vi "_Save_data.vi"(0 "vihlp Path":path, 7 "Info extracted from old HTML":T1={"_vi_name_"="", "_vi_description_text_"="", "_vi_controls_and_indicators_descriptions_"="", "_name_of_owning_library_"="", "_owning_library_html_"="", "_Packages_"="Base Package", "_Platforms_"="Windows", "_details_text_"="Put details here", "_example_screenshot_"="", "_example_vi_"="", "_path_to_example_file_"=path "", "IsDetailsON?"=FALSE, "IsOwningLibraryON?"=FALSE, "IsExamplesON?"=FALSE, "IsTableON?"=FALSE, "IsScrollableON?"=FALSE, "IsDetailedHelpLinkON?"=FALSE, "Table Objects array"=[], "Table Descriptions array"=[], "Table Links array"=[], "Start path location"=enum."VI folder"}, 11 "error in":errorcluster) -> (15 "error out":errorcluster)   [LabVIEW 2012]
uses:
  _Controls and TypeDefs/InfoFromOldHTML_cluster.ctl
  _Controls and TypeDefs/StartPathLocation_enum.ctl
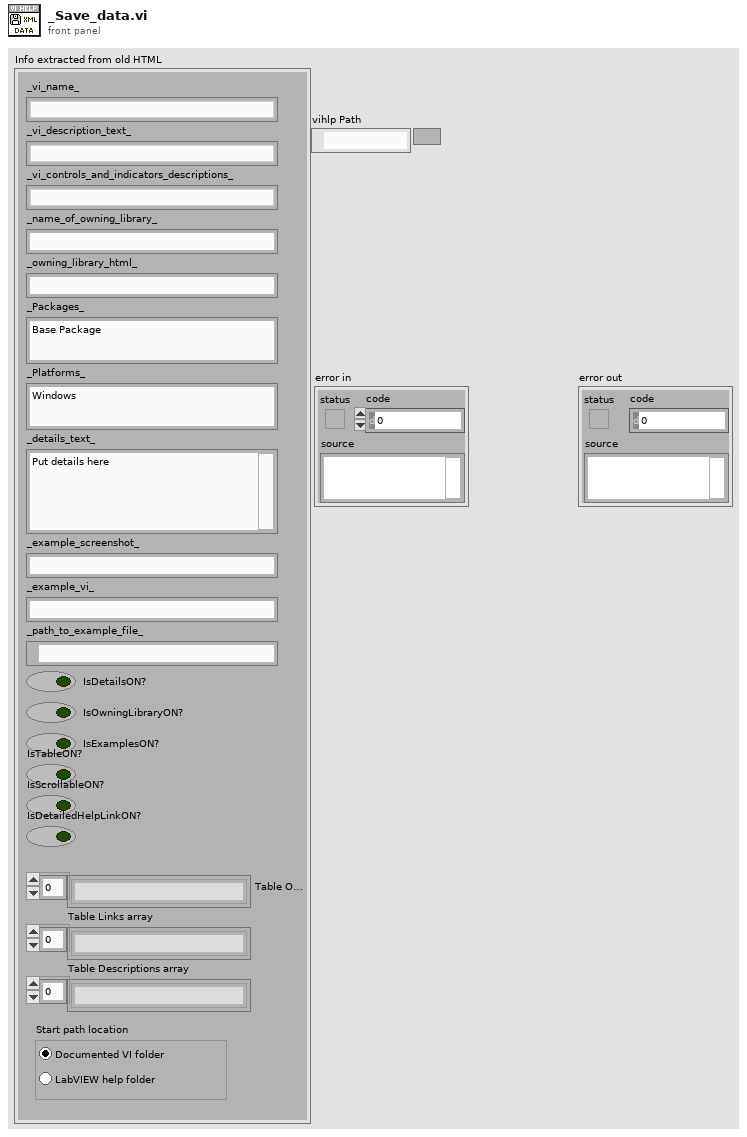
[diagram p1: front panel]
types:
  T1 = typedef "InfoFromOldHTML_cluster.ctl" = cluster{"_vi_name_":string, "_vi_description_text_":string, "_vi_controls_and_indicators_descriptions_":string, "_name_of_owning_library_":string, "_owning_library_html_":string, "_Packages_":string, "_Platforms_":string, "_details_text_":string, "_example_screenshot_":string, "_example_vi_":string, "_path_to_example_file_":path, "IsDetailsON?":bool, "IsOwningLibraryON?":bool, "IsExamplesON?":bool, "IsTableON?":bool, "IsScrollableON?":bool, "IsDetailedHelpLinkON?":bool, "Table Objects array":string[], "Table Descriptions array":string[], "Table Links array":string[], "Start path location":T2}
  T2 = typedef "StartPathLocation_enum.ctl" = enum32{"VI folder", "Help folder"}
  T3 = enum16{"open", "replace", "create", "open or create", "replace or create", "replace or create with confirmation"}
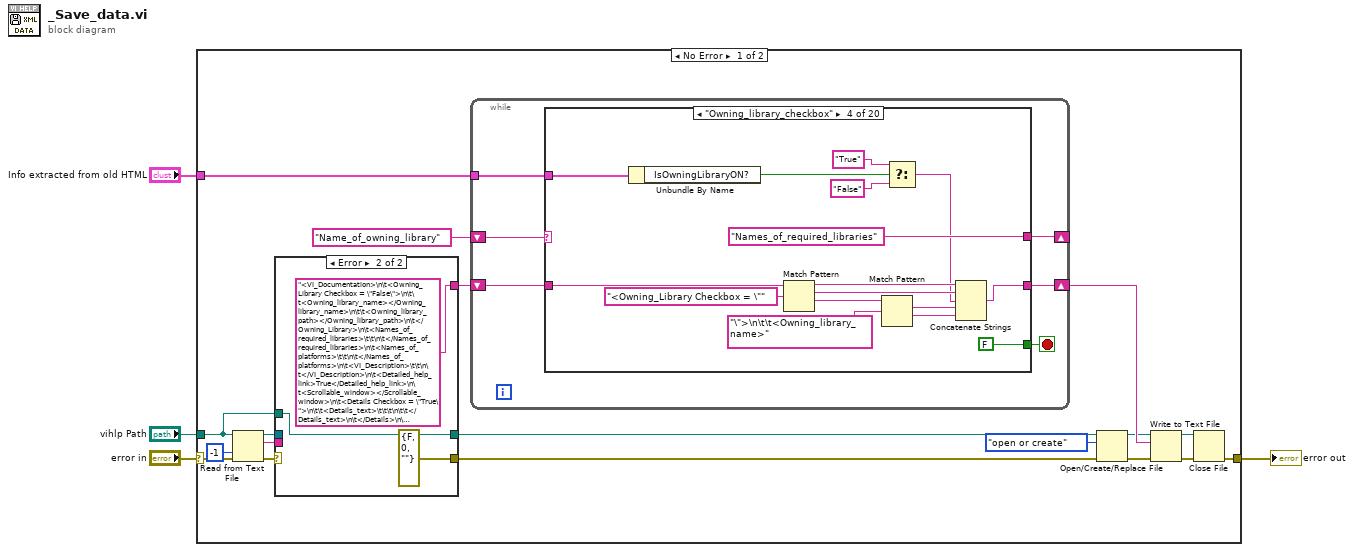
[diagram p0: block diagram]
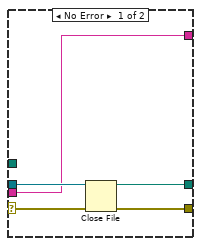
[diagram p2: hidden frame]
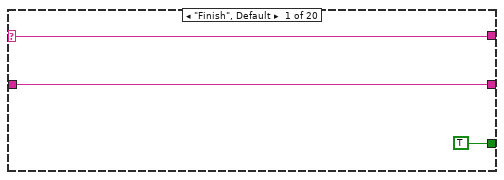
[diagram p3: hidden frame]
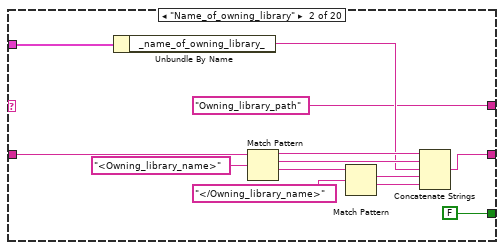
[diagram p4: hidden frame]
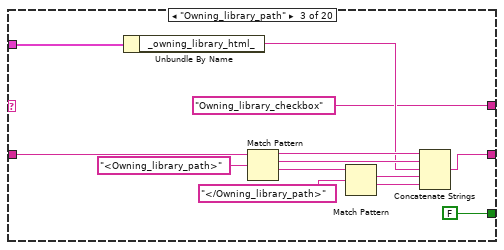
[diagram p5: hidden frame]
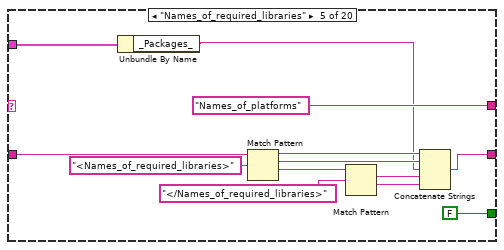
[diagram p6: hidden frame]
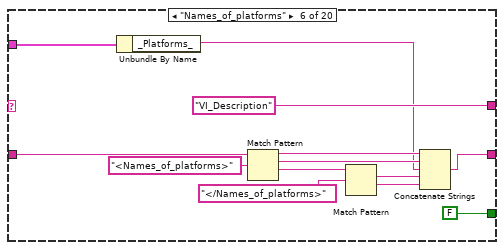
[diagram p7: hidden frame]
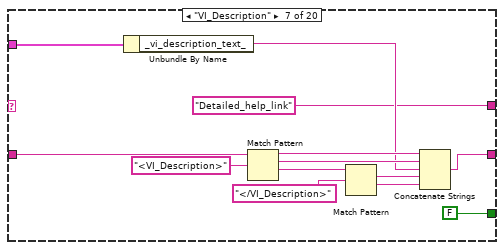
[diagram p8: hidden frame]
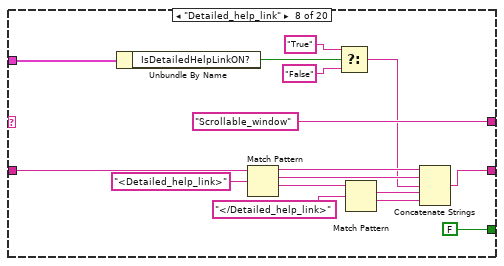
[diagram p9: hidden frame]
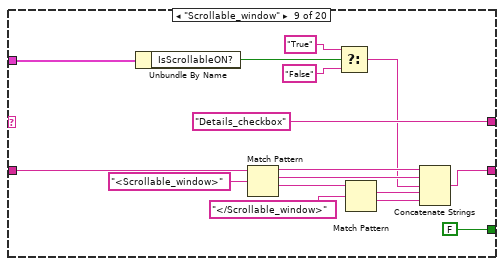
[diagram p10: hidden frame]
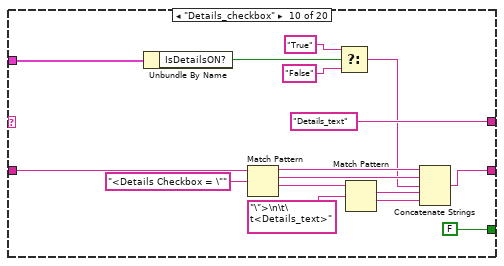
[diagram p11: hidden frame]
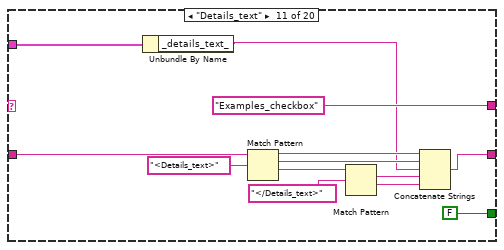
[diagram p12: hidden frame]
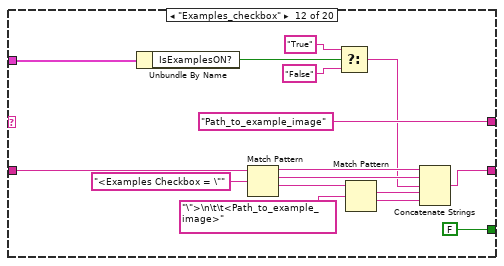
[diagram p13: hidden frame]
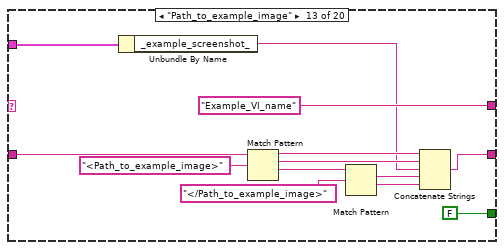
[diagram p14: hidden frame]
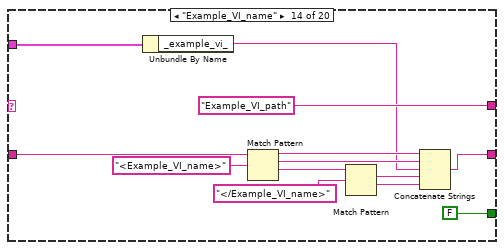
[diagram p15: hidden frame]
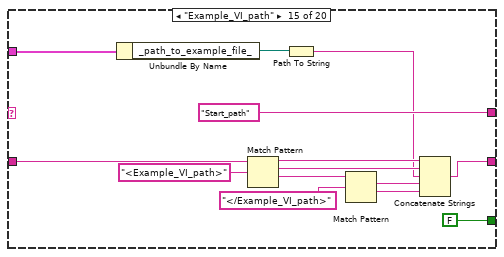
[diagram p16: hidden frame]
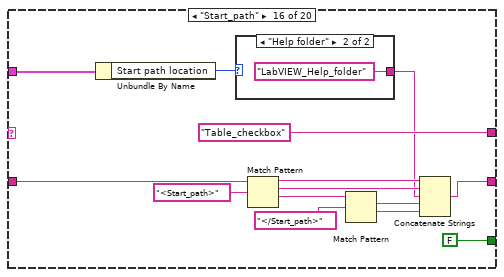
[diagram p17: hidden frame]
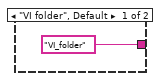
[diagram p18: hidden frame]
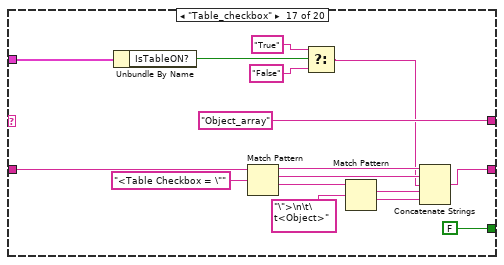
[diagram p19: hidden frame]
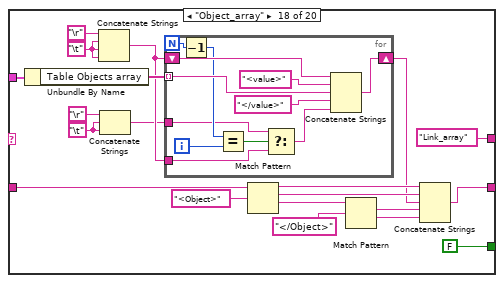
[diagram p20: hidden frame]
diagram:
  n1 = case shown="No Error" "error in" {
    selector: "error in" -> [w5 w366]
    tunnel: "Info extracted from old HTML" -> [w17 _]
    tunnel: [w16 w366] -> w3
    tunnel: "vihlp Path" -> [w11 _]
    frame No Error {
      n2 = Read from Text File(file (use dialog)=w11, count=-1, error in=w5) -> (refnum out=w14:refnum<file>, text=w13:string, error out=w15:errorcluster)  [unwired: 1 in, 1 out]
      n3 = case shown="Error" w15 {
        selector: w15 -> [w27 _]
        tunnel: w14 -> [w26 _]
        tunnel: w13 -> [w25 _]
        tunnel: [w25 "<VI_Documentation>\n\t<Owning_Library Checkbox = \"False\">\n\t\t<Owning_library_name></Owning_library_name>\n\t\t<Owning_library_path></Owning_library_path>\n\t</Owning_Library>\n\t<Names_of_required_libraries>\t\t\n\t</Names_of_required_libraries>\n\t<Names_of_platforms>\t\t\n\t</Names_of_platforms>\n\t<VI_Description>\t\t\n\t</VI_Description>\n\t<Detailed_help_link>True</Detailed_help_link>\n\t<Scrollable_window></Scrollable_window>\n\t<Details Checkbox = \"True\">\n\t\t<Details_text>\t\t\t\n\t\t</Details_text>\n\t</Details>\n\t<Examples Checkbox = \"False\">\n\t\t<Path_to_example_image></Path_to_example_image>\n\t\t<Example_VI_name></Example_VI_name>\n\t\t<Example_VI_path></Example_VI_path>\t\n\t</Examples>\n\t<Start_path>VI_Folder</Start_path>\n\t<Table Checkbox = \"False\">\n\t\t<Object>\n\t\t\t<value></value>\n\t\t</Object>\n\t\t<Link>\n\t\t\t<value></value>\n\t\t</Link>\n\t\t<Description>\n\t\t\t<value></value>\n\t\t</Description>\n\t</Table>\t\n</VI_Documentation>"] -> w12
        tunnel: [w24 errorcluster {"status"=FALSE, "code"=0, "source"=""} ("error constant")] -> w9
        tunnel: [w23 w30] -> w10
        tunnel: w11 -> [_ w30]
        frame No Error {
          n4 = Close File(refnum=w26, error in=w27) -> (path=w23:path, error out=w24:errorcluster)
        }
        frame Error {
        }
      }
      n5 = while {
        shift-right: [w35] -> w19
        shift-left: w12 -> [w36]
        shift-right: [w32] -> _
        shift-left: "Name_of_owning_library" -> [w34]
        tunnel: w17 -> [w33]
        stop <- w31 stop-if-true
        n6 = case shown="\"Owning_library_checkbox\"" w34 {
          selector: w34 -> [w38 _ _ _ _ _ _ _ _ _ _ _ _ _ _ _ _ _ _ _]
          tunnel: w36 -> [w37 w42 w55 w72 w85 w98 w116 w132 w148 w164 w177 w193 w206 w219 w233 w247 w265 w285 w317 w349]
          tunnel: [w37 w41 w54 w71 w84 w97 w112 w128 w144 w160 w173 w189 w202 w215 w229 w243 w261 w281 w313 w345] -> w35
          tunnel: w33 -> [_ w51 w64 w80 w93 w106 w111 w127 w143 w159 w172 w188 w201 w214 w228 w242 w260 w280 w312 w344]
          tunnel: [w38 "Owning_library_path" "Owning_library_checkbox" "Names_of_required_libraries" "Names_of_platforms" "VI_Description" "Detailed_help_link" "Scrollable_window" "Details_checkbox" "Details_text" "Examples_checkbox" "Path_to_example_image" "Example_VI_name" "Example_VI_path" "Start_path" "Table_checkbox" "Object_array" "Link_array" "Description_array" "Finish"] -> w32
          tunnel: [TRUE FALSE FALSE FALSE FALSE FALSE FALSE FALSE FALSE FALSE FALSE FALSE FALSE FALSE FALSE FALSE FALSE FALSE FALSE FALSE] -> w31
          frame "Finish", Default {
          }
          frame "Name_of_owning_library" {
            n7 = Unbundle By Name(w51) -> ("_name_of_owning_library_"=w43:string)
            n8 = Match Pattern(string=w42, regular expression="<Owning_library_name>") -> (before substring=w47:string, match substring=w46:string, after substring=w49:string)  [unwired: 1 in, 1 out]
            n9 = Match Pattern(string=w49, regular expression="</Owning_library_name>") -> (match substring=w44:string, after substring=w45:string)  [unwired: 1 in, 2 out]
            n10 = Concatenate Strings(w47, w46, w43, w44, w45) -> (w41:string)
          }
          frame "Owning_library_path" {
            n11 = Unbundle By Name(w64) -> ("_owning_library_html_"=w56:string)
            n12 = Match Pattern(string=w55, regular expression="<Owning_library_path>") -> (before substring=w60:string, match substring=w59:string, after substring=w62:string)  [unwired: 1 in, 1 out]
            n13 = Match Pattern(string=w62, regular expression="</Owning_library_path>") -> (match substring=w57:string, after substring=w58:string)  [unwired: 1 in, 2 out]
            n14 = Concatenate Strings(w60, w59, w56, w57, w58) -> (w54:string)
          }
          frame "Owning_library_checkbox" {
            n15 = Unbundle By Name(w80) -> ("IsOwningLibraryON?"=w69:bool)
            n16 = Match Pattern(string=w72, regular expression="<Owning_Library Checkbox = \"") -> (before substring=w76:string, match substring=w75:string, after substring=w78:string)  [unwired: 1 in, 1 out]
            n17 = Match Pattern(string=w78, regular expression="\">\n\t\t<Owning_library_name>") -> (match substring=w73:string, after substring=w74:string)  [unwired: 1 in, 2 out]
            n18 = Select(t="True", s=w69, f="False") -> (s? t:f=w67:string)
            n19 = Concatenate Strings(w76, w75, w67, w73, w74) -> (w71:string)
          }
          frame "Names_of_required_libraries" {
            n20 = Unbundle By Name(w93) -> ("_Packages_"=w82:string)
            n21 = Match Pattern(string=w85, regular expression="<Names_of_required_libraries>") -> (before substring=w89:string, match substring=w88:string, after substring=w91:string)  [unwired: 1 in, 1 out]
            n22 = Match Pattern(string=w91, regular expression="</Names_of_required_libraries>") -> (match substring=w86:string, after substring=w87:string)  [unwired: 1 in, 2 out]
            n23 = Concatenate Strings(w89, w88, w82, w86, w87) -> (w84:string)
          }
          frame "Names_of_platforms" {
            n24 = Unbundle By Name(w106) -> ("_Platforms_"=w95:string)
            n25 = Match Pattern(string=w98, regular expression="<Names_of_platforms>") -> (before substring=w102:string, match substring=w101:string, after substring=w104:string)  [unwired: 1 in, 1 out]
            n26 = Match Pattern(string=w104, regular expression="</Names_of_platforms>") -> (match substring=w99:string, after substring=w100:string)  [unwired: 1 in, 2 out]
            n27 = Concatenate Strings(w102, w101, w95, w99, w100) -> (w97:string)
          }
          frame "VI_Description" {
            n28 = Unbundle By Name(w111) -> ("_vi_description_text_"=w110:string)
            n29 = Match Pattern(string=w116, regular expression="<VI_Description>") -> (before substring=w117:string, match substring=w115:string, after substring=w119:string)  [unwired: 1 in, 1 out]
            n30 = Match Pattern(string=w119, regular expression="</VI_Description>") -> (match substring=w113:string, after substring=w114:string)  [unwired: 1 in, 2 out]
            n31 = Concatenate Strings(w117, w115, w110, w113, w114) -> (w112:string)
          }
          frame "Detailed_help_link" {
            n32 = Unbundle By Name(w127) -> ("IsDetailedHelpLinkON?"=w122:bool)
            n33 = Match Pattern(string=w132, regular expression="<Detailed_help_link>") -> (before substring=w133:string, match substring=w131:string, after substring=w135:string)  [unwired: 1 in, 1 out]
            n34 = Select(t="True", s=w122, f="False") -> (s? t:f=w121:string)
            n35 = Match Pattern(string=w135, regular expression="</Detailed_help_link>") -> (match substring=w129:string, after substring=w130:string)  [unwired: 1 in, 2 out]
            n36 = Concatenate Strings(w133, w131, w121, w129, w130) -> (w128:string)
          }
          frame "Scrollable_window" {
            n37 = Unbundle By Name(w143) -> ("IsScrollableON?"=w138:bool)
            n38 = Match Pattern(string=w148, regular expression="<Scrollable_window>") -> (before substring=w149:string, match substring=w147:string, after substring=w151:string)  [unwired: 1 in, 1 out]
            n39 = Select(t="True", s=w138, f="False") -> (s? t:f=w137:string)
            n40 = Match Pattern(string=w151, regular expression="</Scrollable_window>") -> (match substring=w145:string, after substring=w146:string)  [unwired: 1 in, 2 out]
            n41 = Concatenate Strings(w149, w147, w137, w145, w146) -> (w144:string)
          }
          frame "Details_checkbox" {
            n42 = Unbundle By Name(w159) -> ("IsDetailsON?"=w154:bool)
            n43 = Match Pattern(string=w164, regular expression="<Details Checkbox = \"") -> (before substring=w165:string, match substring=w163:string, after substring=w167:string)  [unwired: 1 in, 1 out]
            n44 = Select(t="True", s=w154, f="False") -> (s? t:f=w153:string)
            n45 = Match Pattern(string=w167, regular expression="\">\n\t\t<Details_text>") -> (match substring=w161:string, after substring=w162:string)  [unwired: 1 in, 2 out]
            n46 = Concatenate Strings(w165, w163, w153, w161, w162) -> (w160:string)
          }
          frame "Details_text" {
            n47 = Unbundle By Name(w172) -> ("_details_text_"=w169:string)
            n48 = Match Pattern(string=w177, regular expression="<Details_text>") -> (before substring=w178:string, match substring=w176:string, after substring=w180:string)  [unwired: 1 in, 1 out]
            n49 = Match Pattern(string=w180, regular expression="</Details_text>") -> (match substring=w174:string, after substring=w175:string)  [unwired: 1 in, 2 out]
            n50 = Concatenate Strings(w178, w176, w169, w174, w175) -> (w173:string)
          }
          frame "Examples_checkbox" {
            n51 = Unbundle By Name(w188) -> ("IsExamplesON?"=w183:bool)
            n52 = Match Pattern(string=w193, regular expression="<Examples Checkbox = \"") -> (before substring=w194:string, match substring=w192:string, after substring=w196:string)  [unwired: 1 in, 1 out]
            n53 = Select(t="True", s=w183, f="False") -> (s? t:f=w182:string)
            n54 = Match Pattern(string=w196, regular expression="\">\n\t\t<Path_to_example_image>") -> (match substring=w190:string, after substring=w191:string)  [unwired: 1 in, 2 out]
            n55 = Concatenate Strings(w194, w192, w182, w190, w191) -> (w189:string)
          }
          frame "Path_to_example_image" {
            n56 = Unbundle By Name(w201) -> ("_example_screenshot_"=w198:string)
            n57 = Match Pattern(string=w206, regular expression="<Path_to_example_image>") -> (before substring=w207:string, match substring=w205:string, after substring=w209:string)  [unwired: 1 in, 1 out]
            n58 = Match Pattern(string=w209, regular expression="</Path_to_example_image>") -> (match substring=w203:string, after substring=w204:string)  [unwired: 1 in, 2 out]
            n59 = Concatenate Strings(w207, w205, w198, w203, w204) -> (w202:string)
          }
          frame "Example_VI_name" {
            n60 = Unbundle By Name(w214) -> ("_example_vi_"=w211:string)
            n61 = Match Pattern(string=w219, regular expression="<Example_VI_name>") -> (before substring=w220:string, match substring=w218:string, after substring=w222:string)  [unwired: 1 in, 1 out]
            n62 = Match Pattern(string=w222, regular expression="</Example_VI_name>") -> (match substring=w216:string, after substring=w217:string)  [unwired: 1 in, 2 out]
            n63 = Concatenate Strings(w220, w218, w211, w216, w217) -> (w215:string)
          }
          frame "Example_VI_path" {
            n64 = Unbundle By Name(w228) -> ("_path_to_example_file_"=w225:path)
            n65 = Match Pattern(string=w233, regular expression="<Example_VI_path>") -> (before substring=w234:string, match substring=w232:string, after substring=w236:string)  [unwired: 1 in, 1 out]
            n66 = Path To String(path=w225) -> (string=w224:string)
            n67 = Match Pattern(string=w236, regular expression="</Example_VI_path>") -> (match substring=w230:string, after substring=w231:string)  [unwired: 1 in, 2 out]
            n68 = Concatenate Strings(w234, w232, w224, w230, w231) -> (w229:string)
          }
          frame "Start_path" {
            n69 = Unbundle By Name(w242) -> ("Start path location"=w239:T2)
            n70 = case shown="\"Help folder\"" w239 {
              tunnel: ["VI_folder" "LabVIEW_Help_folder"] -> w238
              frame "VI folder", Default {
              }
              frame "Help folder" {
              }
            }
            n71 = Match Pattern(string=w247, regular expression="<Start_path>") -> (before substring=w248:string, match substring=w246:string, after substring=w250:string)  [unwired: 1 in, 1 out]
            n72 = Match Pattern(string=w250, regular expression="</Start_path>") -> (match substring=w244:string, after substring=w245:string)  [unwired: 1 in, 2 out]
            n73 = Concatenate Strings(w248, w246, w238, w244, w245) -> (w243:string)
          }
          frame "Table_checkbox" {
            n74 = Unbundle By Name(w260) -> ("IsTableON?"=w255:bool)
            n75 = Match Pattern(string=w265, regular expression="<Table Checkbox = \"") -> (before substring=w266:string, match substring=w264:string, after substring=w268:string)  [unwired: 1 in, 1 out]
            n76 = Select(t="True", s=w255, f="False") -> (s? t:f=w254:string)
            n77 = Match Pattern(string=w268, regular expression="\">\n\t\t<Object>") -> (match substring=w262:string, after substring=w263:string)  [unwired: 1 in, 2 out]
            n78 = Concatenate Strings(w266, w264, w254, w262, w263) -> (w261:string)
          }
          frame "Object_array" {
            w272 = "\t"
            w275 = "\t"
            n79 = Unbundle By Name(w280) -> ("Table Objects array"=w277:string[])
            n80 = Concatenate Strings("\r", w275, w275, w275) -> (w271:string)
            n81 = Concatenate Strings("\r", w272, w272) -> (w270:string)
            n82 = for {
              N -> [w297]
              tunnel: w277 -> [w300] mode=indexing
              shift-right: [w298] -> w274
              shift-left: w271 -> [w299]
              tunnel: w271 -> [w292]
              tunnel: w270 -> [w291]
              i -> [w295]
              n83 = Decrement(x=w297) -> (x-1=w296:i32)
              n84 = Equal?(x=w296, y=w295) -> (x = y?=w293:bool)
              n85 = Select(t=w291, s=w293, f=w292) -> (s? t:f=w290:string)
              n86 = Concatenate Strings(w299, "<value>" ("regular expression"), w300, "</value>" ("regular expression"), w290) -> (w298:string)
            }
            n87 = Match Pattern(string=w285, regular expression="<Object>") -> (before substring=w286:string, match substring=w284:string, after substring=w288:string)  [unwired: 1 in, 1 out]
            n88 = Match Pattern(string=w288, regular expression="</Object>") -> (match substring=w282:string, after substring=w283:string)  [unwired: 1 in, 2 out]
            n89 = Concatenate Strings(w286, w284, w274, w282, w283) -> (w281:string)
          }
          frame "Link_array" {
            w304 = "\t"
            w307 = "\t"
            n90 = Unbundle By Name(w312) -> ("Table Links array"=w309:string[])
            n91 = Concatenate Strings("\r", w307, w307, w307) -> (w303:string)
            n92 = Concatenate Strings("\r", w304, w304) -> (w302:string)
            n93 = for {
              N -> [w328]
              tunnel: w309 -> [w332] mode=indexing
              shift-right: [w329] -> w306
              shift-left: w303 -> [w330]
              tunnel: w303 -> [w324]
              tunnel: w302 -> [w323]
              i -> [w326]
              n94 = Decrement(x=w328) -> (x-1=w327:i32)
              n95 = Equal?(x=w327, y=w326) -> (x = y?=w325:bool)
              n96 = Select(t=w323, s=w325, f=w324) -> (s? t:f=w322:string)
              n97 = Concatenate Strings(w330, "<value>" ("regular expression"), w332, "</value>" ("regular expression"), w322) -> (w329:string)
            }
            n98 = Match Pattern(string=w317, regular expression="<Link>") -> (before substring=w318:string, match substring=w316:string, after substring=w320:string)  [unwired: 1 in, 1 out]
            n99 = Match Pattern(string=w320, regular expression="</Link>") -> (match substring=w314:string, after substring=w315:string)  [unwired: 1 in, 2 out]
            n100 = Concatenate Strings(w318, w316, w306, w314, w315) -> (w313:string)
          }
          frame "Description_array" {
            w335 = "\t"
            w339 = "\t"
            n101 = Unbundle By Name(w344) -> ("Table Descriptions array"=w341:string[])
            n102 = Concatenate Strings("\r", w339, w339, w339) -> (w337:string)
            n103 = Concatenate Strings("\r", w335, w335) -> (w334:string)
            n104 = for {
              N -> [w360]
              tunnel: w341 -> [w364] mode=indexing
              shift-right: [w362] -> w338
              shift-left: w337 -> [w363]
              tunnel: w337 -> [w356]
              tunnel: w334 -> [w354]
              i -> [w361]
              n105 = Decrement(x=w360) -> (x-1=w359:i32)
              n106 = Equal?(x=w359, y=w361) -> (x = y?=w357:bool)
              n107 = Select(t=w354, s=w357, f=w356) -> (s? t:f=w355:string)
              n108 = Concatenate Strings(w363, "<value>" ("regular expression"), w364, "</value>" ("regular expression"), w355) -> (w362:string)
            }
            n109 = Match Pattern(string=w349, regular expression="<Description>") -> (before substring=w350:string, match substring=w348:string, after substring=w352:string)  [unwired: 1 in, 1 out]
            n110 = Match Pattern(string=w352, regular expression="</Description>") -> (match substring=w346:string, after substring=w347:string)  [unwired: 1 in, 2 out]
            n111 = Concatenate Strings(w350, w348, w338, w346, w347) -> (w345:string)
          }
        }
      }
      n112 = Open/Create/Replace File(file path (use dialog)=w10, error in=w9, operation (0:open)=T3."open or create") -> (refnum out=w8:refnum<file>, error out=w7:errorcluster)  [unwired: 3 in, 1 out]
      n113 = Write to Text File(file (use dialog)=w8, text=w19, error in=w7) -> (refnum out=w22:refnum<file>, error out=w21:errorcluster)  [unwired: 1 in, 1 out]
      n114 = Close File(refnum=w22, error in=w21) -> (error out=w16:errorcluster)  [unwired: 1 out]
    }
    frame Error {
    }
  }
  "error out" <- w3
